vi "date_path_h5.vi"(7 "Bases":path[](array[path]), 9 "SEQ File":path caption="SEQ File (*.osq)", 10 "time stamp":timestamp) -> (1 "RID":string, 2 "H5":path[](array[path]))   [LabVIEW 2013]
uses:
  <vilib>/addons/h5labview2/file/H5Fmode.ctl
  <vilib>/addons/h5labview2/base/lib_path.vi
  <vilib>/addons/h5labview2/base/H5Equery.vi
  <vilib>/addons/h5labview2/attrib/H5Awrite.llb/H5Awrite.xnode
  <vilib>/addons/h5labview2/file/H5F.lvlib
panel:
  out "error out":errorcluster
  in  "error in":errorcluster
  in  "Save":bool=TRUE
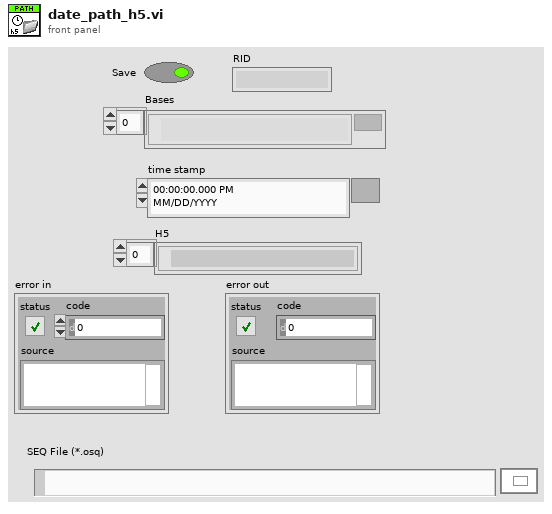
[diagram p1: front panel]
types:
  T1 = typedef "H5F.lvlib/H5Fmode.ctl" = enum16{"read-only", "read-write", "overwrite", "create new", "open or create"}
  T2 = typedef "hid_t.ctl" = i32
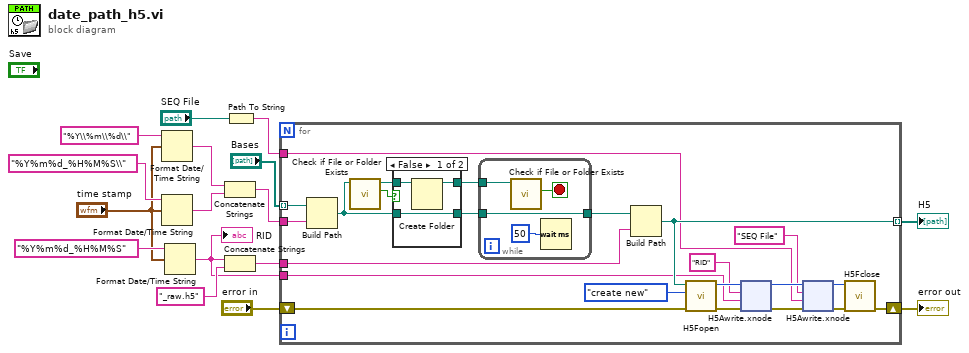
[diagram p0: block diagram]
diagram:
  n1 = Format Date/Time String(time format string (%c)="%Y\\%m\\%d\\", seconds (now)="time stamp") -> (date/time string=w15:string)  [unwired: 1 in]
  n2 = Format Date/Time String(time format string (%c)="%Y%m%d_%H%M%S\\", seconds (now)="time stamp") -> (date/time string=w12:string)  [unwired: 1 in]
  n3 = Format Date/Time String(time format string (%c)="%Y%m%d_%H%M%S", seconds (now)="time stamp") -> (date/time string=w3:string)  [unwired: 1 in]
  "RID" <- w3
  n4 = Concatenate Strings(w15, w12) -> (w14:string)
  n5 = Concatenate Strings(w3, "_raw.h5" ("string")) -> (w6:string)
  n6 = Path To String(path="SEQ File") -> (string=w1:string)
  n7 = for {
    tunnel: w14 -> [w39]
    tunnel: "Bases" -> [w34] mode=indexing
    tunnel: [w29] -> w8 mode=indexing
    tunnel: w6 -> [w31]
    shift-right: [w28] -> w4
    shift-left: "error in" -> [w27]
    tunnel: w3 -> [w24]
    tunnel: w1 -> [w18]
    n8 = Build Path(base path=w34, name or relative path=w39) -> (appended path=w33:path)
    n9 = call <vilib>:"Check if File or Folder Exists.vi"("path"=w33) -> ("file or folder exists?"=w38:bool, "dup path"=w37:path)  [unwired: 8 in, 1 out]
    n10 = case shown="False" w38 {
      tunnel: w37 -> [w82 w83]
      tunnel: [w81 w84] -> w35
      tunnel: w33 -> [w81 w84]
      tunnel: [w80 w83] -> w36
      frame False {
        n11 = Create Folder(path (use dialog)=w82) -> (created path=w80:path)  [unwired: 2 in, 2 out]
      }
      frame True {
      }
    }
    n12 = while {
      tunnel: w36 -> [w78]
      tunnel: [w76] -> w32
      tunnel: w35 -> [w76]
      stop <- w79 stop-if-true
      n13 = call <vilib>:"Check if File or Folder Exists.vi"("path"=w78) -> ("file or folder exists?"=w79:bool)  [unwired: 8 in, 2 out]
      n14 = Wait (ms)(milliseconds to wait=u32 50) -> ()  [unwired: 1 out]
    }
    n15 = Build Path(base path=w32, name or relative path=w31) -> (appended path=w29:path)
    n16 = call <vilib>:"H5Fopen.vi"("error in (no error)"=w27, "mode (read-only)"=H5Fmode."create new", "path"=w29) -> ("error out"=w26:errorcluster, "ref out"=w25:T2)  [unwired: 7 in]
    n17 = xnode "H5Awrite.xnode"("error in (no error)"=w26, "data"=w24, "attrib name"="RID", "ref in"=w25) -> ("error out"=w20:errorcluster, "ref out"=w22:i32)  [unwired: 3 in, 1 out]
    n18 = xnode "H5Awrite.xnode"("error in (no error)"=w20, "data"=w18, "attrib name"="SEQ File", "ref in"=w22) -> ("error out"=w19:errorcluster, "ref out"=w21:i32)  [unwired: 3 in, 1 out]
    n19 = call <vilib>:"H5Fclose.vi"("error in (no error)"=w19, "ref"=w21) -> ("error out"=w28:errorcluster)  [unwired: 9 in]
  }
  "H5" <- w8
  "error out" <- w4
